vi "model config var.vi"() -> ()   [LabVIEW 2022 SP3, in "斯坦道总磷总氮.lvlib"]
panel:
  out "启动队列名称":cluster{"String":string, "Value":u16}[](array[cluster])
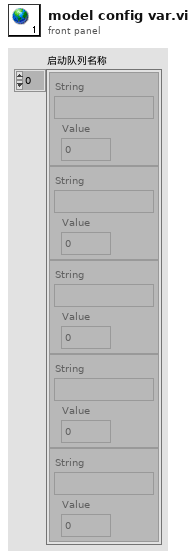
[diagram p1: front panel]
diagram:
